vi "init.vi"(8 "error in (no error)":errorcluster, 11 "StepperMotor in":refnum<class "StepperMotor.lvclass">) -> (0 "error out":errorcluster, 3 "StepperMotor out":refnum<class "StepperMotor.lvclass">)   [LabVIEW 2013, in "StepperMotor.lvclass"]
uses:
  StepperMotor.lvclass
  Configuration/Stepper Motor.ctl
  StepperMotor.lvclass/StepperMotor.ctl
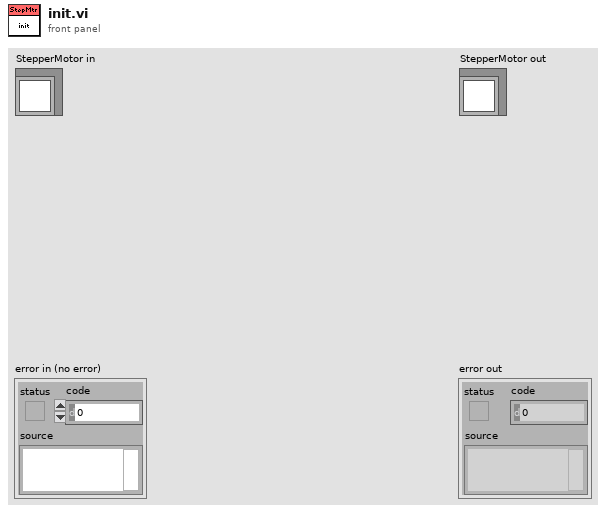
[diagram p1: front panel]
types:
  T1 = typedef "Stepper Motor.ctl" = cluster{"Maximum Step Rate":dbl[unit]}
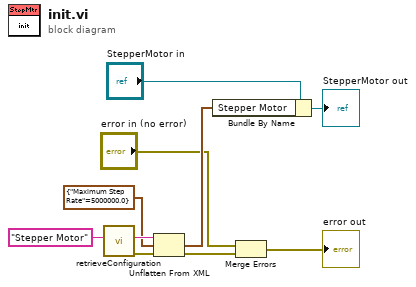
[diagram p0: block diagram]
diagram:
  n1 = call "retrieveConfiguration.vi"("configName"="Stepper Motor") -> ("error out"=w7:errorcluster, "xmlData"=w6:string)  [unwired: 9 in]
  n2 = Unflatten From XML(xml string=w6, type=T1 {"Maximum Step Rate"=5000000.0} ("Stepper Motor"), error in (no error)=w7) -> (value=w10:T1, error out=w9:errorcluster)
  n3 = Bundle By Name(cluster="StepperMotor in", "Stepper Motor"=w10) -> (→"StepperMotor out":refnum<class "StepperMotor.lvclass">)
  n4 = Merge Errors("error in (no error)", w9) -> (→"error out":errorcluster)
